vi "FGV.vi"(8 "error in":errorcluster, 10 "DB Item":T1 {"Balance" format="%#.2g"}, 11 "Mode":T3) -> (0 "error out":errorcluster, 3 "Defaults":T2 {"Records"."Balance" format="%#.2g"})   [LabVIEW 2020, in "Configuration Database.lvlib"]
doc: "Internal Reference holder for Database"
uses:
  Configuration Database.lvlib
  Controls/FGV Mode.ctl
  Controls/FGV Data.ctl
  Controls/DB item.ctl
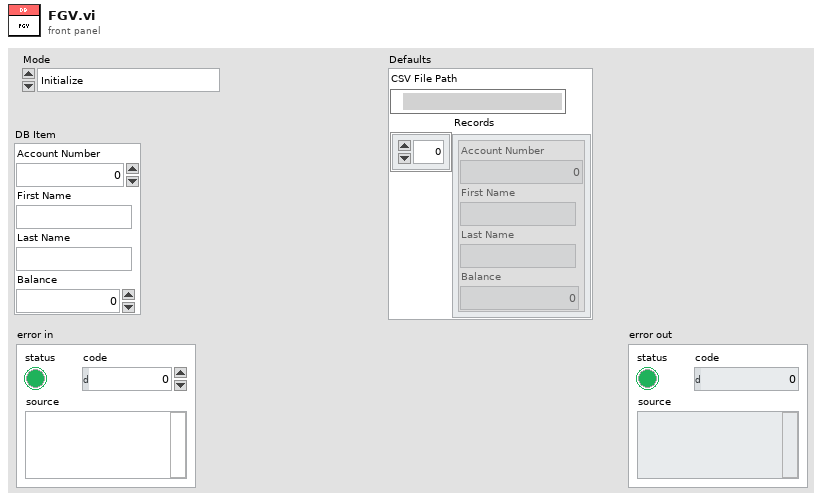
[diagram p1: front panel]
types:
  T1 = typedef "Configuration Database.lvlib/DB item.ctl" = cluster{"Account Number":i32, "First Name":string, "Last Name":string, "Balance":dbl}
  T2 = typedef "Configuration Database.lvlib/FGV Data.ctl" = cluster{"CSV File Path":path, "Records":T1[]}
  T3 = typedef "Configuration Database.lvlib/FGV Mode.ctl" = enum16{"Initialize", "Get", "Set"}
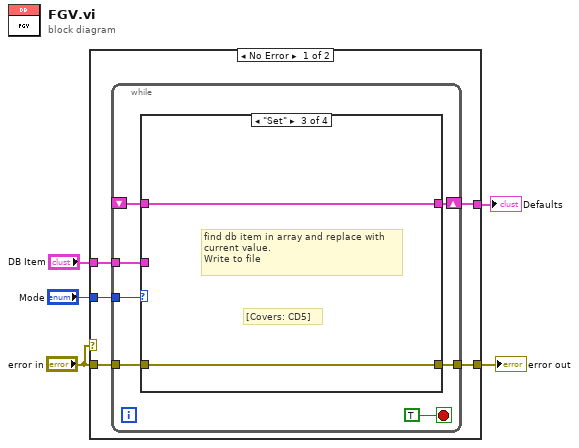
[diagram p0: block diagram]
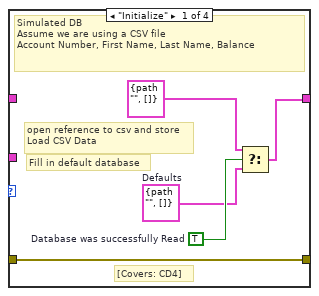
[diagram p2: hidden frame]
diagram:
  n1 = case shown="No Error" "error in" {
    tunnel: [w10 w29] -> w5
    tunnel: "error in" -> [w9 w29]
    tunnel: "Mode" -> [w8 _]
    tunnel: [w7 _] -> w2
    tunnel: "DB Item" -> [w6 _]
    frame No Error {
      n2 = while {
        tunnel: [w17] -> w10
        tunnel: w9 -> [w16]
        tunnel: w8 -> [w14]
        shift-right: [w12] -> w7
        shift-left: _ -> [w13]
        tunnel: w6 -> [w11]
        stop <- TRUE stop-if-true
        n3 = case shown="\"Set\"" w14 {
          tunnel: [w22 w24 w26 w28] -> w17
          tunnel: w16 -> [w22 w24 w26 w28]
          tunnel: w13 -> [_ w23 w25 w27]
          tunnel: [w18 w23 w25 w27] -> w12
          tunnel: w11 -> [_ _ _ _]
          frame "Initialize" {
            w21 = TRUE  # Database was successfully Read
            w20 = T2 {"CSV File Path"=path "", "Records"=[]}  # Defaults
            # "[Covers: CD4]"
            # "Fill in default database"
            # "open reference to csv and store\nLoad CSV Data"
            # "Simulated DB\nAssume we are using a CSV file\nAccount Number, First Name, Last Name, Balance"
            n4 = Select(t=T2 {"CSV File Path"=path "", "Records"=[]} ("FGV Data"), s=w21, f=w20) -> (s? t:f=w18:T2)
          }
          frame "Get" {
          }
          frame "Set" {
            # "[Covers: CD5]"
            # "find db item in array and replace with\ncurrent value.\nWrite to file"
          }
          frame Default {
          }
        }
      }
    }
    frame Error {
    }
  }
  "error out" <- w5
  "Defaults" <- w2
